vi "MSEncoder SubVI WfmCodeAccess_AuxScan.vi"(8 "error in":errorcluster, 10 "Data in":T2={"Wfm type"=2, "Start conj #"=2, "TotalAuxCyc#"=3.0, "mz0"=880.97278970104787987, "Scan rate"=-33305.06819671684353, "MathieuEqParame"={"mz(Th)"=747.75251691418050576, "Amp(V)"=330.0, "Freq(Hz)"=199999.99552965164, "Beta"=0.8, "r_0 (mm)"=7.07106781187, "z_0 (mm)"=10.0}, "Amp0"=1.0, "Amp ramp rate"=-0.0, "Pulse1 Amp"=1.0, "Pulse2 Amp"=-1.0, "Scan time"=0.0039999999999999999998, "Beta scale"=1.0} {"MathieuEqParame"."Freq(Hz)" format="%#_2g"; "MathieuEqParame"."Amp(V)" format="%#.2g"; "MathieuEqParame"."mz(Th)" format="%#.2g"}, 11 "MSEncoder in":refnum<class "MSEncoder.lvclass">) -> (0 "error out":errorcluster, 3 "MSEncoder out":refnum<class "MSEncoder.lvclass">)   [LabVIEW 2018, in "MSEncoder.lvclass"]
uses:
  MSEncoder.lvclass
  PublicSubVI/Ctl/MathieuEqParam.ctl
  MSEncoder.lvclass/MSEncoder.ctl
  WfmDataAccessor/WfmDataAccessor.lvclass
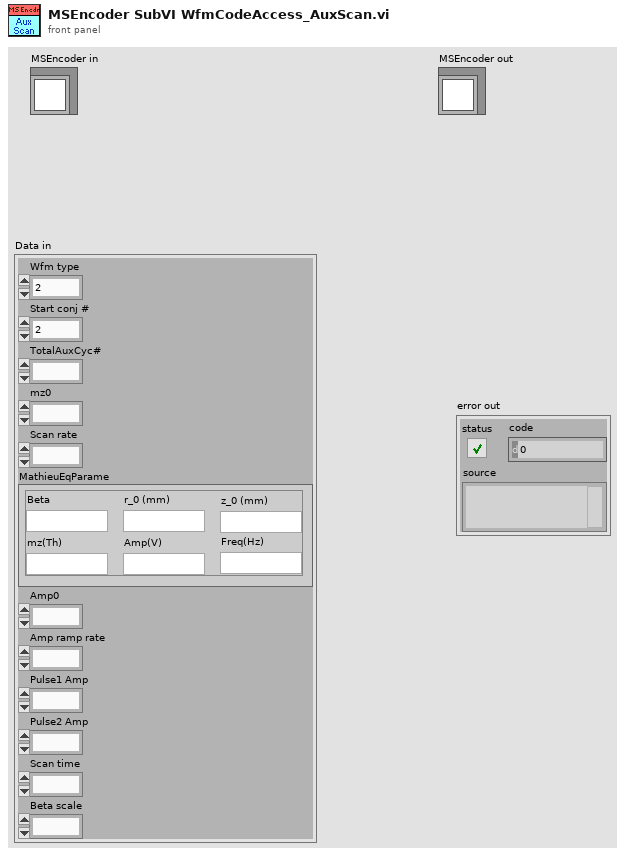
[diagram p1: front panel]
types:
  T1 = typedef "MathieuEqParam.ctl" = cluster{"mz(Th)":ext, "Amp(V)":ext, "Freq(Hz)":ext, "Beta":ext, "r_0 (mm)":ext, "z_0 (mm)":ext}
  T2 = cluster{"Wfm type":u64, "Start conj #":u32, "TotalAuxCyc#":ext, "mz0":ext, "Scan rate":ext, "MathieuEqParame":T1, "Amp0":ext, "Amp ramp rate":ext, "Pulse1 Amp":ext, "Pulse2 Amp":ext, "Scan time":ext, "Beta scale":ext}
  T3 = cluster{"Data in":cluster{"Wfm type":u64, "Start conj #":u32, "TotalAuxCyc#":ext, "mz0":ext, "Scan rate":ext, "MathieuEqParame":T1, "Amp0":ext, "Amp ramp rate":ext, "Pulse1 Amp":ext, "Pulse2 Amp":ext, "Scan time":ext, "Beta scale":ext}, "CycDiff":u64[], "Ratio":u16[], "1/Decyc":u32, "Decyc":u32}
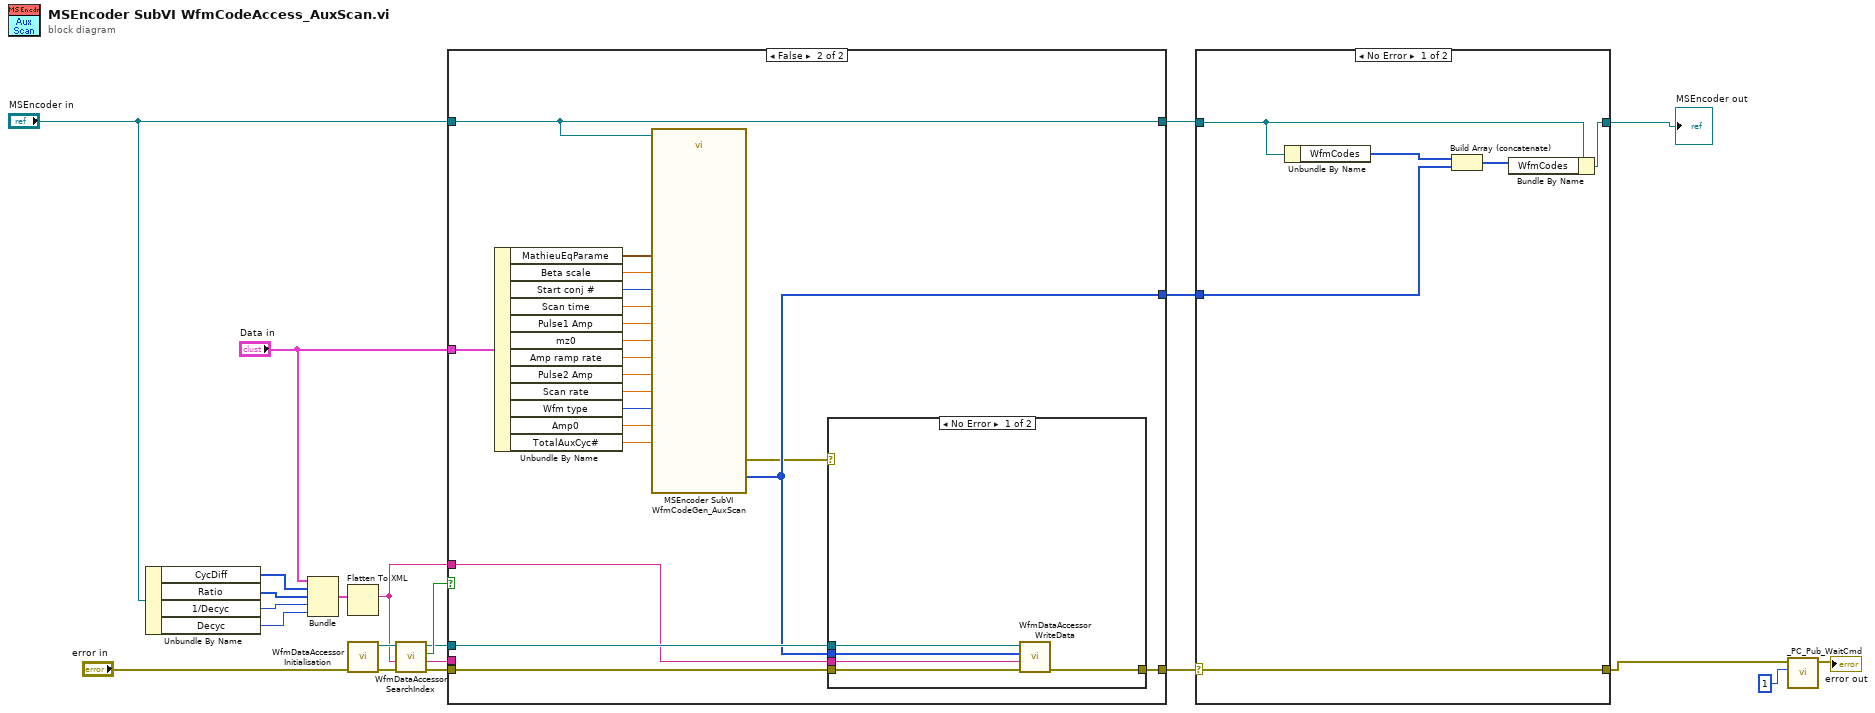
[diagram p0: block diagram]
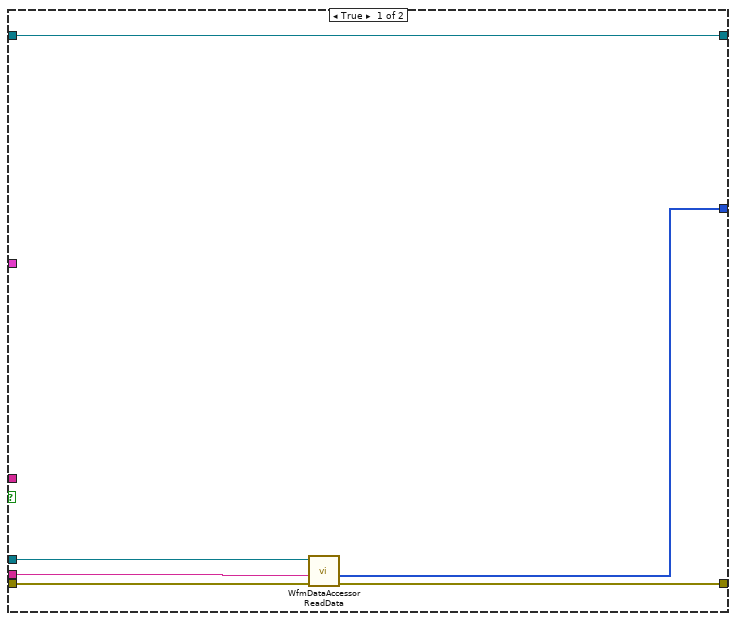
[diagram p3: hidden frame]
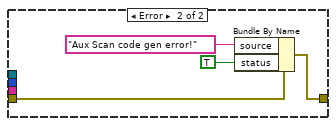
[diagram p4: hidden frame]
diagram:
  n1 = Unbundle By Name("MSEncoder in") -> ("CycDiff"=w19:u64[], "Ratio"=w20:u16[], "1/Decyc"=w21:u32, "Decyc"=w22:u32)
  n2 = Bundle("Data in"="Data in", "CycDiff"=w19, "Ratio"=w20, "1/Decyc"=w21, "Decyc"=w22) -> (w18:T3)  [unwired: 1 in]
  n3 = Flatten To XML(anything=w18) -> (xml string=w10:string)
  n4 = call "WfmDataAccessor Initialisation.vi"("error in (no error)"="error in") -> ("error out"=w9:errorcluster, "WfmDataAccessor out"=w11:refnum<class "WfmDataAccessor.lvclass">)  [unwired: 9 in]
  n5 = call-dynamic "WfmDataAccessor SearchIndex.vi"("error in (no error)"=w9, "XML in"=w10, "WfmDataAccessor in"=w11) -> ("error out"=w6:errorcluster, "filename"=w5:string, "Found"=w8:bool, "WfmDataAccessor out"=w7:refnum<class "WfmDataAccessor.lvclass">)  [unwired: 5 in]
  n6 = case shown="False" w8 {
    tunnel: [w23 w46] -> w17
    tunnel: "MSEncoder in" -> [w28 w48]
    tunnel: "Data in" -> [_ w44]
    tunnel: [w24 w45] -> w13
    tunnel: w10 -> [_ w29]
    tunnel: [w28 w48] -> w14
    tunnel: w7 -> [w27 w47]
    tunnel: w6 -> [w25 w36]
    tunnel: w5 -> [w26 _]
    frame True {
      n7 = call-dynamic "WfmDataAccessor ReadData.vi"("error in (no error)"=w25, "Filename"=w26, "WfmDataAccessor in"=w27) -> ("error out"=w24:errorcluster, "WfmData"=w23:u64[])  [unwired: 6 in, 1 out]
    }
    frame False {
      n8 = Unbundle By Name(w44) -> ("MathieuEqParame"=w43:T1, "Beta scale"=w41:ext, "Start conj #"=w42:u32, "Scan time"=w40:ext, "Pulse1 Amp"=w39:ext, "mz0"=w38:ext, "Amp ramp rate"=w37:ext, "Pulse2 Amp"=w35:ext, "Scan rate"=w34:ext, "Wfm type"=w33:u64, "Amp0"=w32:ext, "TotalAuxCyc#"=w31:ext)
      n9 = call "MSEncoder SubVI WfmCodeGen_AuxScan.vi"("MSEncoder in"=w48, "Scan time"=w40, "Pulse1 Amp"=w39, "mz0"=w38, "Amp ramp rate"=w37, "Pulse2 Amp"=w35, "Start conj #"=w42, "Scan rate"=w34, "Beta scale"=w41, "Wfm type"=w33, "MathieuEqParame"=w43, "Amp0"=w32, "TotalAuxCyc#"=w31) -> ("WfmCode"=w46:u64[], "error out"=w30:errorcluster)  [unwired: 5 in]
      n10 = case shown="No Error" w30 {
        tunnel: w47 -> [w53 _]
        tunnel: w46 -> [w52 _]
        tunnel: w29 -> [w51 _]
        tunnel: [w50 w56] -> w45
        tunnel: w36 -> [w49 w57]
        frame No Error {
          n11 = call-dynamic "WfmDataAccessor WriteData.vi"("error in (no error)"=w49, "XML"=w51, "WfmData"=w52, "WfmDataAccessor in"=w53) -> ("error out"=w50:errorcluster)  [unwired: 6 in, 1 out]
        }
        frame Error {
          n12 = Bundle By Name(cluster=w57, "source"="Aux Scan code gen error!", "status"=TRUE) -> (w56:errorcluster)
        }
      }
    }
  }
  n13 = case shown="No Error" w13 {
    selector: w13 -> [w59 w65]
    tunnel: [w62 w64] -> w3
    tunnel: w14 -> [w61 w64]
    tunnel: w17 -> [w60 _]
    tunnel: [w59 w65] -> w12
    frame No Error {
      n14 = Unbundle By Name(w61) -> ("WfmCodes"=w63:u64[])
      n15 = Build Array (concatenate)(w63, w60) -> (w58:u64[])
      n16 = Bundle By Name(cluster=w61, "WfmCodes"=w58) -> (w62:refnum<class "MSEncoder.lvclass">)
    }
    frame Error {
    }
  }
  "MSEncoder out" <- w3
  n17 = call "_PC_Pub_WaitCmd.vi"("milliseconds to wait"=u32 1, "error in (no error)"=w12) -> ("error out"=→"error out":errorcluster)  [unwired: 9 in]
